vi "_Validate Path.vi"(1 "Check Type (F)":bool, 2 "Check Exist (F)":bool, 3 "Type (isd)":string="isd", 4 "path":path) -> (0 "Valid":bool)   [LabVIEW 2018, in "Function Lib.lvlib"]
doc: "Check if the path of file name is valid."
uses:
  Function Lib.lvlib
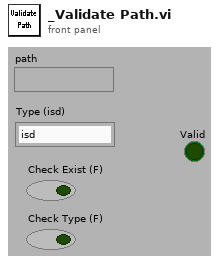
[diagram p1: front panel]
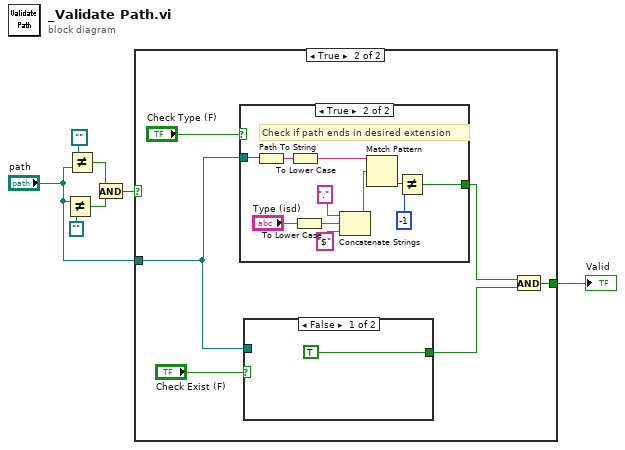
[diagram p0: block diagram]
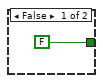
[diagram p2: hidden frame]
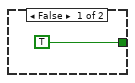
[diagram p3: hidden frame]
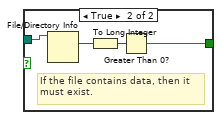
[diagram p4: hidden frame]
diagram:
  n1 = Not Equal?(x="path", y=path "") -> (x != y?=w7:bool)
  n2 = Not Equal?(x=path "", y="path") -> (x != y?=w6:bool)
  n3 = And(x=w6, y=w7) -> (x .and. y?=w3:bool)
  n4 = case shown="True" w3 {
    tunnel: "path" -> [_ w9]
    tunnel: [FALSE w10] -> w1
    frame False {
    }
    frame True {
      n5 = case shown="True" "Check Type (F)" {
        tunnel: [TRUE w18] -> w12
        tunnel: w9 -> [_ w23]
        frame False {
        }
        frame True {
          # "Check if path ends in desired extension"
          n6 = Path To String(path=w23) -> (string=w22:string)
          n7 = To Lower Case(string=w22) -> (all lower case string=w17:string)
          n8 = To Lower Case(string="Type (isd)") -> (all lower case string=w16:string)
          n9 = Concatenate Strings("." ("Substring"), w16, "$" ("Substring")) -> (w21:string)
          n10 = Match Pattern(string=w17, regular expression=w21) -> (offset past match=w20:i32)  [unwired: 4 out]
          n11 = Not Equal?(x=w20, y=-1) -> (x != y?=w18:bool)
        }
      }
      n12 = case shown="False" "Check Exist (F)" {
        tunnel: [TRUE w31] -> w11
        tunnel: w9 -> [_ w30]
        frame False {
          (unwired) TRUE
        }
        frame True {
          # "If the file contains data, then it \nmust exist."
          n13 = File/Directory Info(path=w30) -> (size=w28:i64)  [unwired: 1 in, 6 out]
          n14 = To Long Integer(number=w28) -> (32bit integer=w29:i32)
          n15 = Greater Than 0?(x=w29) -> (x > 0?=w31:bool)
        }
      }
      n16 = And(x=w12, y=w11) -> (x .and. y?=w10:bool)
    }
  }
  "Valid" <- w1
